vi "Open.vi"   [LabVIEW 2013]
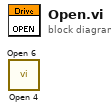
[diagram p0: block diagram]
diagram:
  n1 = call "Open 4.vi"() -> ()  [unwired: 10 in, 2 out]
  n2 = call "Open 6.vi"() -> ()  [unwired: 10 in, 2 out]
